vi "Close.vi"(8 "error in (no error)":errorcluster, 11 "FLOM Settings in":T1) -> (0 "error out":errorcluster, 1 "Connection Error":bool, 3 "FLOM Settings out":T1)   [LabVIEW 2021, in "FLOM Pump.lvlib"]
uses:
  FLOM Pump.lvlib
  Settings Cluster.ctl
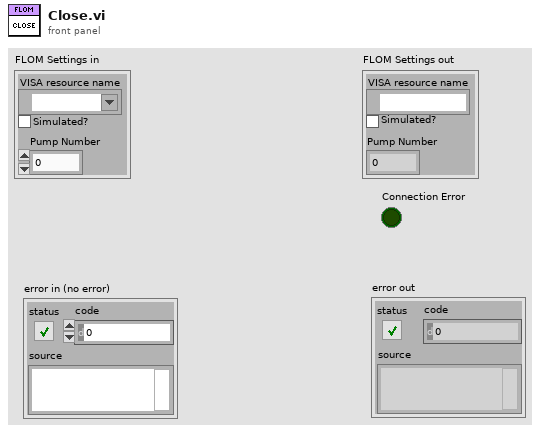
[diagram p1: front panel]
types:
  T1 = typedef "FLOM Pump.lvlib/Settings Cluster.ctl" = cluster{"VISA resource name":refnum<visa-resource-name>, "Simulated?":bool, "Pump Number":dbl}
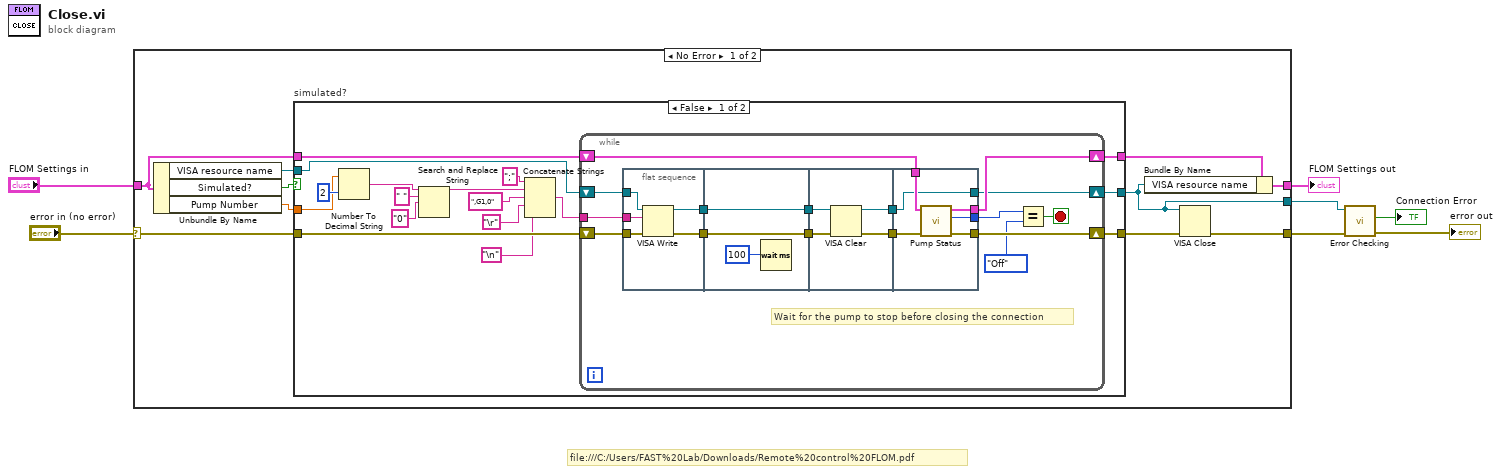
[diagram p0: block diagram]
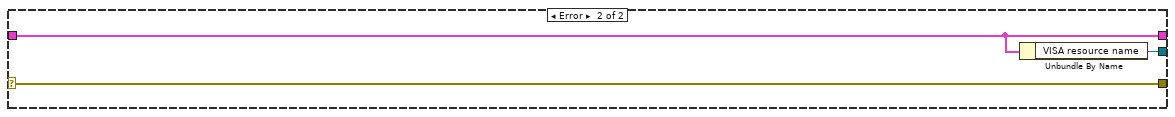
[diagram p3: hidden frame]
diagram:
  # "file:///C:/Users/FAST%20Lab/Downloads/Remote%20control%20FLOM.pdf"
  n1 = case shown="No Error" "error in (no error)" {
    selector: "error in (no error)" -> [w14 w74]
    tunnel: [w9 w74] -> w2
    tunnel: [w16 w73] -> w5
    tunnel: "FLOM Settings in" -> [w12 w73]
    tunnel: [w8 w72] -> w3
    frame No Error {
      n2 = Unbundle By Name(w12) -> ("VISA resource name"=w13:refnum<visa-resource-name>, "Simulated?"=w17:bool, "Pump Number"=w15:dbl)
      n3 = case "simulated?" shown="False" w17 {
        tunnel: [w34 w70] -> w10
        tunnel: [w26 w69] -> w8
        tunnel: w15 -> [w19 _]
        tunnel: w14 -> [w30 w70]
        tunnel: w13 -> [w25 w69]
        tunnel: w12 -> [w28 w71]
        tunnel: [w27 w71] -> w11
        frame False {
          n4 = Number To Decimal String(number=w19, width (-)=i16 2) -> (decimal integer string=w22:string)
          n5 = Search and Replace String(input string=w22, search string=" ", replace string="0" ("replace string (\"\")")) -> (result string=w18:string)  [unwired: 5 in, 3 out]
          n6 = Concatenate Strings(";" ("string"), w18, ",G1,0" ("string"), "\r", "\n") -> (w29:string)
          n7 = while {
            tunnel: w29 -> [w43]
            shift-right: [w45] -> w34
            shift-left: w30 -> [w44]
            shift-right: [w41] -> w27
            shift-left: w28 -> [w42]
            shift-right: [w40] -> w26
            shift-left: w25 -> [w38]
            stop <- w36 stop-if-true
            # "Wait for the pump to stop before closing the connection"
            n8 = flat-sequence {
              tunnel: [w51] -> w50
              tunnel: [w52] -> w49
              tunnel: w44 -> [w55]
              tunnel: w43 -> [w54]
              tunnel: w38 -> [w53]
              tunnel: [w58] -> w48
              tunnel: [w57] -> w47
              tunnel: w50 -> [w58]
              tunnel: w49 -> [w57]
              tunnel: w48 -> [w62]
              tunnel: w47 -> [w61]
              tunnel: [w60] -> w46
              tunnel: [w59] -> w39
              tunnel: [w67] -> w45
              tunnel: w46 -> [w68]
              tunnel: w42 -> [w66]
              tunnel: [w65] -> w41
              tunnel: [w64] -> w37
              tunnel: [w63] -> w40
              tunnel: w39 -> [w63]
              frame #0 {
                n9 = VISA Write(VISA resource name=w53, write buffer=w54, error in (no error)=w55) -> (VISA resource name out=w51:refnum<visa-resource-name>, error out=w52:errorcluster)  [unwired: 1 out]
              }
              frame #1 {
                n10 = Wait (ms)(milliseconds to wait=u32 100) -> ()  [unwired: 1 out]
              }
              frame #2 {
                n11 = VISA Clear(VISA resource name=w62, error in (no error)=w61) -> (VISA resource name out=w59:refnum<visa-resource-name>, error out=w60:errorcluster)
              }
              frame #3 {
                n12 = call "Pump Status.vi"("error in (no error)"=w68, "FLOM Settings In"=w66) -> ("error out"=w67:errorcluster, "Pump On?"=w64:enum16{"Off", "On", "Not Initialized"}, "FLOM Settings Out"=w65:T1)  [unwired: 4 in, 3 out]
              }
            }
            n13 = Equal?(x=w37, y=enum16{"Off", "On", "Not Initialized"}."Off") -> (x = y?=w36:bool)
          }
        }
        frame True {
        }
      }
      n14 = Bundle By Name(cluster=w11, "VISA resource name"=w8) -> (w16:T1)
      n15 = VISA Close(VISA resource name=w8, error in (no error)=w10) -> (error out=w9:errorcluster)
    }
    frame Error {
      n16 = Unbundle By Name(w73) -> ("VISA resource name"=w72:refnum<visa-resource-name>)
    }
  }
  "FLOM Settings out" <- w5
  n17 = call "Error Checking.vi"("error in (no error)"=w2, "VISA resource name"=w3) -> ("error out"=→"error out":errorcluster, "Connection Error"=→"Connection Error":bool)  [unwired: 7 in, 1 out]
